vi "Control_signals_VI.vi"(6 "Input":T1(ring)=enum."Zero State (Omron)", 7 "error in":errorcluster) -> (1 "Current Mode":string, 2 "error out":errorcluster)   [LabVIEW 2020]
panel:
  in  "Increase Pressure":cluster{"CTRL A":dbl, "CTRL B":dbl}={"CTRL A"=0.0, "CTRL B"=5.0}
  in  "Reduce Pressure":cluster{"CTRL A":dbl, "CTRL B":dbl}={"CTRL A"=5.0, "CTRL B"=5.0}
  in  "Hold Pressure":cluster{"CTRL A":dbl, "CTRL B":dbl}={"CTRL A"=5.0, "CTRL B"=0.0}
  in  "Zero State":cluster{"CTRL A":dbl, "CTRL B":dbl}
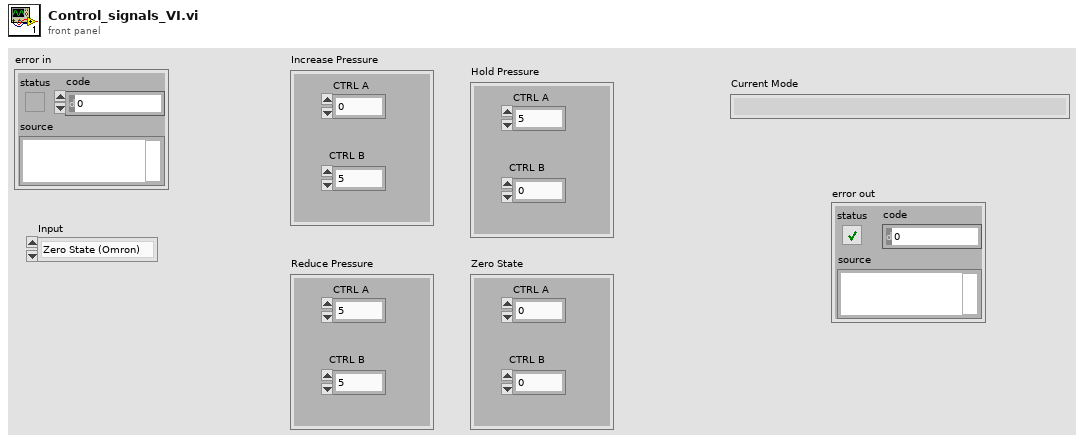
[diagram p1: front panel]
types:
  T1 = enum16{"Increase Pressure", "Reduce Pressure", "Hold Pressure", "Zero State (Omron)"}
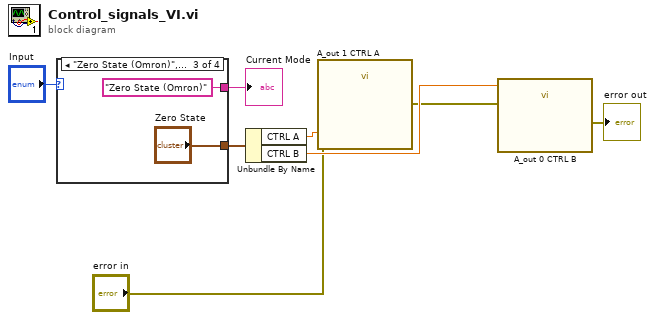
[diagram p0: block diagram]
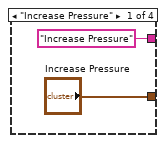
[diagram p2: hidden frame]
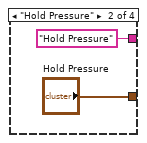
[diagram p3: hidden frame]
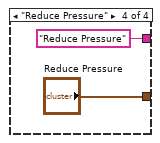
[diagram p4: hidden frame]
diagram:
  n1 = case shown="\"Zero State (Omron)\", Default" "Input" {
    tunnel: ["Increase Pressure" "Hold Pressure" "Zero State" "Reduce Pressure"] -> w3
    tunnel: ["Increase Pressure" "Hold Pressure" "Zero State (Omron)" "Reduce Pressure"] -> w2
    frame "Increase Pressure" {
    }
    frame "Hold Pressure" {
    }
    frame "Zero State (Omron)", Default {
    }
    frame "Reduce Pressure" {
    }
  }
  "Current Mode" <- w2
  n2 = Unbundle By Name(w3) -> ("CTRL A"=w7:dbl, "CTRL B"=w8:dbl)
  n3 = call "A_out 1 CTRL A"("data"=w7, "error in"="error in") -> ("error out"=w5:errorcluster)  [unwired: 16 in, 1 out]
  n4 = call "A_out 0 CTRL B"("data"=w8, "error in"=w5) -> ("error out"=→"error out":errorcluster)  [unwired: 16 in, 1 out]
